vi "发送指令.vi"(3 "C":string="0", 4 "Y":string="0", 5 "X":string="0") -> (2 "发送指令":string)   [LabVIEW 2016]
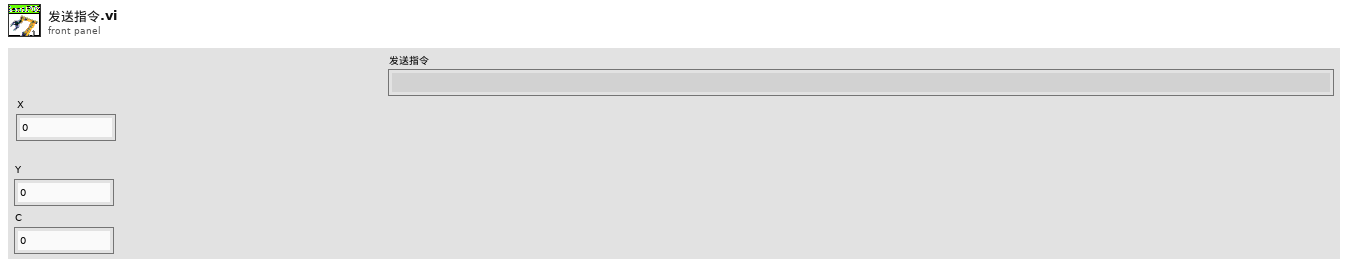
[diagram p1: front panel]
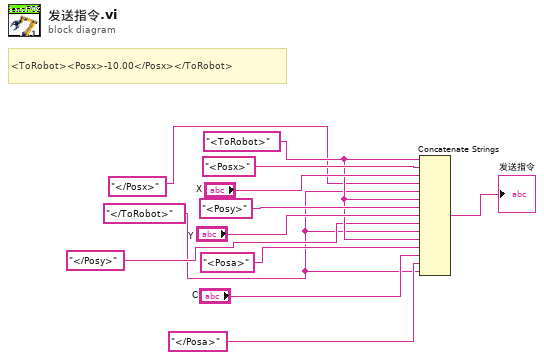
[diagram p0: block diagram]
diagram:
  w1 = "</ToRobot>"
  w5 = "<ToRobot>"
  # "<ToRobot><Posx>-10.00</Posx></ToRobot>"
  n1 = Concatenate Strings(w5, "<Posx>", "X", "</Posx>", w1, w5, "<Posy>", "Y", "</Posy>", w1, w5, "<Posa>", "C", "</Posa>", w1) -> (→"发送指令":string)
